vi "Open Mag Cal file.vi"(0 "Magnet Id":string) -> (1 "String":string, 2 "Error":bool, 3 "Error Code":i32, 4 "Error message":string)   [LabVIEW 2024]
uses:
  <vilib>/Utility/error.llb/DialogType.ctl
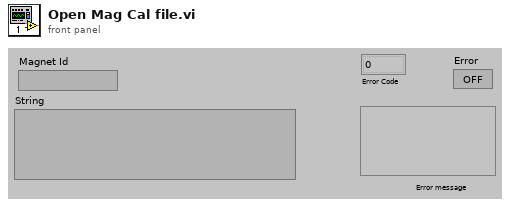
[diagram p1: front panel]
types:
  T1 = typedef "DialogType.ctl" = u16
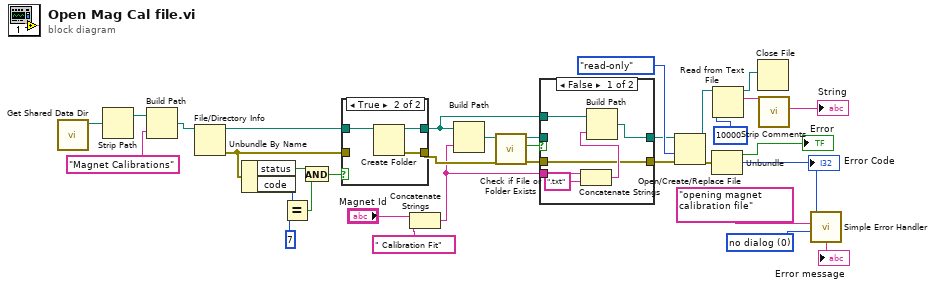
[diagram p0: block diagram]
diagram:
  w15 = T1 0 items=["no dialog", "OK message", "continue or stop message", "OK message + warnings", "continue/stop + warnings"] ("type of dialog (OK msg:1)")
  n1 = call "Get Shared Data Dir.vi"() -> ("Data Directory Path"=w3:path)  [unwired: 2 in, 1 out]
  n2 = Strip Path(path=w3) -> (stripped path=w4:path)  [unwired: 1 out]
  n3 = Build Path(base path=w4, name or relative path="Magnet Calibrations") -> (appended path=w1:path)
  n4 = File/Directory Info(path=w1) -> (path out=w16:path, error out=w22:errorcluster)  [unwired: 1 in, 5 out]
  n5 = Unbundle By Name(w22) -> ("status"=w19:bool, "code"=w21:i32)
  n6 = Equal?(x=w21, y=7) -> (x = y?=w18:bool)
  n7 = And(x=w19, y=w18) -> (x .and. y?=w17:bool)
  n8 = case shown="True" w17 {
    tunnel: w16 -> [w35 w39]
    tunnel: [w35 w38] -> w8
    tunnel: [w36 w37] -> w12
    tunnel: w22 -> [w36 _]
    frame False {
    }
    frame True {
      n9 = Create Folder(path (use dialog)=w39) -> (created path=w38:path, error out=w37:errorcluster)  [unwired: 2 in, 1 out]
    }
  }
  n10 = Concatenate Strings("Magnet Id", " Calibration Fit") -> (w7:string)
  n11 = Build Path(base path=w8, name or relative path=w7) -> (appended path=w13:path)
  n12 = call <vilib>:"Check if File or Folder Exists.vi"("error in (no error)"=w12, "path"=w13) -> ("error out"=w10:errorcluster, "file or folder exists?"=w11:bool, "dup path"=w9:path)  [unwired: 7 in]
  n13 = case shown="False" w11 {
    tunnel: w10 -> [w41 w46]
    tunnel: w9 -> [_ w47]
    tunnel: w8 -> [w45 _]
    tunnel: w7 -> [w43 _]
    tunnel: [w40 w47] -> w6
    tunnel: [w41 w46] -> w5
    frame False {
      n14 = Concatenate Strings(w43, ".txt" ("string")) -> (w44:string)
      n15 = Build Path(base path=w45, name or relative path=w44) -> (appended path=w40:path)
    }
    frame True {
    }
  }
  n16 = Open/Create/Replace File(file path (use dialog)=w6, error in=w5, access (0:read/write)=enum16{"read/write", "read-only", "write-only"}."read-only") -> (refnum out=w29:refnum<file>, error out=w31:errorcluster)  [unwired: 3 in, 1 out]
  n17 = Unbundle(w31) -> ("status"=→"Error":bool, "code"=w24:i32)  [unwired: 1 out]
  "Error Code" <- w24
  n18 = Read from Text File(file (use dialog)=w29, count=10000) -> (refnum out=w28:refnum<file>, text=w27:string)  [unwired: 2 in, 2 out]
  n19 = Close File(refnum=w28) -> ()  [unwired: 1 in, 2 out]
  n20 = call "Strip Comments.vi"(1:w27) -> (0:→"String":string)
  n21 = call <vilib>:"Simple Error Handler.vi"("error code (no error:0)"=w24, "error source (\" \")"="opening magnet calibration file", "type of dialog (OK msg:1)"=w15) -> ("message"=→"Error message":string)  [unwired: 2 in, 4 out]
